vi "ProjectInstance.vi"(11 "error in (no error)":errorcluster) -> (15 "error out":errorcluster)   [LabVIEW 2016, in "Drona Test.lvlib"]
uses:
  Drona Test.lvlib
  main/apis/Setup/GetVI/GetVIByPath.vi
  <vilib>/addons/_JKI Toolkits/Caraya/classes/Assert/Assert Not Error.vi
  <vilib>/addons/_JKI Toolkits/Caraya/classes/Assert/Assert.lvclass
  <vilib>/addons/_JKI Toolkits/Caraya/classes/Test/Test.lvclass
  main/Drona.lvlib
  main/apis/Setup/GetVI/GetVI.lvlib
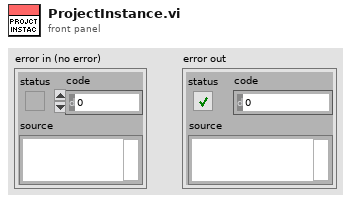
[diagram p1: front panel]
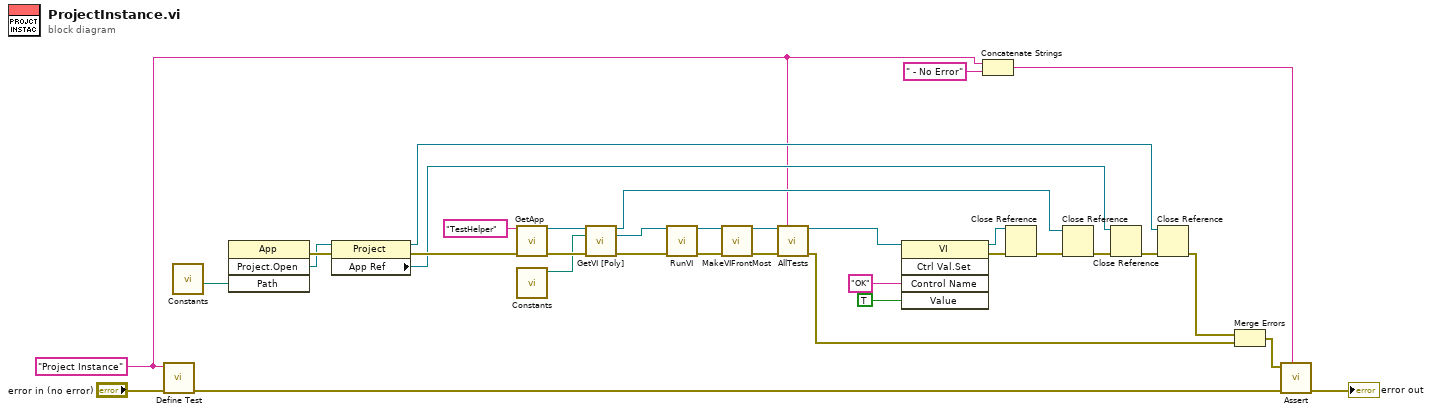
[diagram p0: block diagram]
diagram:
  w1 = "Project Instance" ("Label (VI Title)")
  n1 = call <vilib>:"Define Test.vi"("error in (no error)"="error in (no error)", "Label (VI Title)"=w1) -> ("error out"=w31:errorcluster)  [unwired: 9 in]
  n2 = call "Constants.vi"() -> ("HelperProject path"=w5:path)  [unwired: 9 in, 2 out]
  n3 = invoke class="App" method="Project.Open"("Path"=w5) -> (error out=w20:errorcluster, "Project:Open"=w19:refnum<vi>)  [unwired: 3 in, 2 out]
  n4 = property class="Project"(reference=w19, error in=w20) -> (reference out=w17:refnum<vi>, error out=w18:errorcluster, "App Ref"=w16:refnum<vi>)
  n5 = call "GetApp.vi"("Project Name (\"\": ThisApplication)"="TestHelper" ("Project Name (\"\": ThisApplication)"), "error in (no error)"=w18) -> ("Application Ref"=w22:refnum<vi>, "error out"=w21:errorcluster)  [unwired: 12 in]
  n6 = call "Constants.vi"() -> ("HelperMain path"=w4:path)  [unwired: 9 in, 2 out]
  n7 = call-poly "GetVI [Poly].vi"("Application Ref in"=w22, "VI Path"=w4, "error in (no error)"=w21) -> ("Application Ref out"=w23:refnum<vi>, "VI Reference"=w24:refnum<vi>, "error out"=w25:errorcluster)  [unwired: 10 in]
  n8 = call "RunVI.vi"("VI Reference In"=w24, "error in"=w25) -> ("VI Reference Out"=w14:refnum<vi>, "error out"=w13:errorcluster)  [unwired: 12 in]
  n9 = call "MakeVIFrontMost.vi"("VI Reference In"=w14, "error in"=w13) -> ("VI Reference Out"=w27:refnum<vi>, "error out"=w26:errorcluster)  [unwired: 12 in]
  n10 = call "AllTests.vi"("VI in"=w27, "Label"=w1, "error in (no error)"=w26) -> ("VI out"=w28:refnum<vi>, "error out"=w2:errorcluster)  [unwired: 11 in]
  n11 = invoke class="VI" method="Ctrl Val.Set"(reference=w28, "Control Name"="OK", "Value"=TRUE) -> (reference out=w11:refnum<vi>, error out=w12:errorcluster)  [unwired: 2 in, 3 out]
  n12 = Concatenate Strings(w1, " - No Error" ("Label (VI Title)")) -> (w29:string)
  n13 = Close Reference(reference=w11, error in (no error)=w12) -> (error out=w8:errorcluster)
  n14 = Close Reference(reference=w23, error in (no error)=w8) -> (error out=w6:errorcluster)
  n15 = Close Reference(reference=w16, error in (no error)=w6) -> (error out=w7:errorcluster)
  n16 = Close Reference(reference=w17, error in (no error)=w7) -> (error out=w3:errorcluster)
  n17 = Merge Errors(w3, w2) -> (w34:errorcluster)
  n18 = call-poly <vilib>:"Assert.vi"("Label"=w29, "error in (no error)"=w31, "Not Error?"=w34) -> ("error out"=→"error out":errorcluster)  [unwired: 8 in]
